vi "heater2.vi"(1 "Tin":dbl, 2 "dt (seconds)":dbl, 3 "Current":dbl, 4 "Tamb":dbl) -> (0 "Tout":dbl)   [LabVIEW 2014]
doc: "Simulates a current-controlled cryostat heater element with conductive cooling described by Fourier's Law. Place this in a While Loop with time step <b>dt</b>.\n\n<b>Tin</b> Present sample temperature\n<b>Tout</b> New sample temperature after time <b>dt</b>\n<b>Tamb</b> Coldfinger temperature\n<b>Current</b> Heater current"
panel:
  # "Output temperature"
  # "Reference temperature (K)"
  # "Control current"
  # "Time step (seconds)"
  # "Actual temperature input"
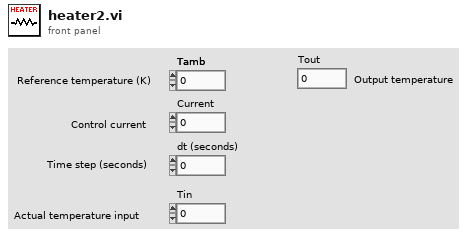
[diagram p1: front panel]
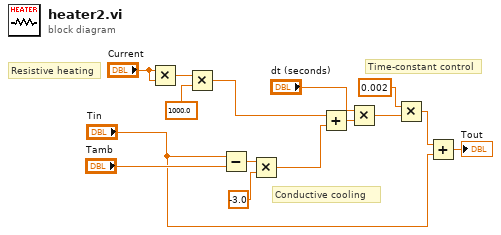
[diagram p0: block diagram]
diagram:
  # "Time-constant control"
  # "Resistive heating"
  # "Conductive cooling"
  n1 = Multiply(x="Current", y="Current") -> (x*y=w14:dbl)
  n2 = Multiply(x=w14, y=1000.0 ("R")) -> (x*y=w9:dbl)
  n3 = Subtract(x="Tin", y="Tamb") -> (x-y=w11:dbl)
  n4 = Multiply(x=w11, y=-3.0) -> (x*y=w8:dbl)
  n5 = Add(x=w9, y=w8) -> (x+y=w4:dbl)
  n6 = Multiply(x="dt (seconds)", y=w4) -> (x*y=w3:dbl)
  n7 = Multiply(x=0.002, y=w3) -> (x*y=w6:dbl)
  n8 = Add(x=w6, y="Tin") -> (x+y=→"Tout":dbl)
